vi "Test Run Asynchronous.vi"(11 "CO2 Settings":T3={"Run C1"={"A-1,  1"=inf, "A-3,  2"=inf, "A-4, 3"=9600.0, "A-5, 4"=8800.0, "ABCD-7, 5"=9800.0, "A-8, 6"=9800.0, "B-1,  7"=3400.0, "B-3, 8"=3400.0, "B-4,  9"=9600.0, "B-5, 10"=8800.0, "B-8, 11"=9800.0, "C-1, 12"=1800.0, "C-3, 13"=1800.0, "C-4, 14"=9600.0, "C-5,  15"=8800.0, "C-8, 16"=9800.0, "D-1, 17"=inf, "D-3, 18"=3400.0, "D-4,  19"=1800.0, "D-5,  20"=9800.0, "D-8,  21"=9800.0}, "Run C2"={"A-1,  1"=inf, "A-3,  2"=inf, "A-4, 3"=9500.0, "A-5, 4"=8600.0, "ABCD-7, 5"=9700.0, "A-8, 6"=9700.0, "B-1,  7"=3000.0, "B-3, 8"=3000.0, "B-4,  9"=9500.0, "B-5, 10"=8600.0, "B-8, 11"=9700.0, "C-1, 12"=1400.0, "C-3, 13"=1400.0, "C-4, 14"=9500.0, "C-5,  15"=8600.0, "C-8, 16"=9700.0, "D-1, 17"=inf, "D-3, 18"=3000.0, "D-4,  19"=1400.0, "D-5,  20"=9700.0, "D-8,  21"=9700.0}, "Hold C3"={"A-1,  1"=1800.0, "A-3,  2"=1800.0, "A-4, 3"=9000.0, "A-5, 4"=8800.0, "ABCD-7, 5"=9800.0, "A-8, 6"=9800.0, "B-1,  7"=3400.0, "B-3, 8"=3400.0, "B-4,  9"=9000.0, "B-5, 10"=8800.0, "B-8, 11"=9800.0, "C-1, 12"=1800.0, "C-3, 13"=1800.0, "C-4, 14"=9000.0, "C-5,  15"=8800.0, "C-8, 16"=9800.0, "D-1, 17"=1800.0, "D-3, 18"=3400.0, "D-4,  19"=1800.0, "D-5,  20"=9800.0, "D-8,  21"=9800.0}, "Hold C4"={"A-1,  1"=1400.0, "A-3,  2"=1400.0, "A-4, 3"=8800.0, "A-5, 4"=8600.0, "ABCD-7, 5"=9700.0, "A-8, 6"=9700.0, "B-1,  7"=3000.0, "B-3, 8"=3000.0, "B-4,  9"=8800.0, "B-5, 10"=8600.0, "B-8, 11"=9700.0, "C-1, 12"=1400.0, "C-3, 13"=1400.0, "C-4, 14"=8800.0, "C-5,  15"=8600.0, "C-8, 16"=9700.0, "D-1, 17"=1400.0, "D-3, 18"=3000.0, "D-4,  19"=1400.0, "D-5,  20"=9700.0, "D-8,  21"=9700.0}, "High CO2 Forces"={"A-1, 1"=TRUE, "A-3, 2"=TRUE, "A-4, 3"=FALSE, "A-5, 4"=TRUE, "ABCD-7, 5"=FALSE, "A-8, 6"=TRUE, "B-1,  7"=TRUE, "B-3, 8"=TRUE, "B-4, 9"=FALSE, "B-5, 10"=TRUE, "B-8,  11"=TRUE, "C-1, 12"=TRUE, "C-3, 13"=TRUE, "C-4,  14"=FALSE, "C-5,  15"=TRUE, "C-8, 16"=TRUE, "D-1, 17"=TRUE, "D-3, 18"=TRUE, "D-4, 19"=TRUE, "D-5,  20"=TRUE, "D-8,  21"=TRUE}}) -> ()   [LabVIEW 2012]
uses:
  Type Defs/AD Settings.ctl
  Type Defs/Output Values.ctl
  Type Defs/Output Switches.ctl
  Type Defs/CO2 Settings.ctl
  Type Defs/Final Output for Dispaly 2.ctl
panel:
  in  "Main Tabs":T1(tab)=enum."CO2 Settings"
  in  "Other Outputs":cluster{"Alarm":bool, "Heater":bool}
  out "CO2 ppm":u32(slide)=493 scale=0.0..10000.0
  out "Alt Dif":dbl(slide)=1604.2180978990014 scale=-1000.0..1000.0 scale format="%.1f"
  out "Final Output":T2
  in  "AD Settings":T6={"Set Point Force"={"A-1,  1"=inf, "A-3,  2"=inf, "A-4, 3"=inf, "A-5, 4"=5790.0, "ABCD-7, 5"=inf, "A-8, 6"=inf, "B-1,  7"=5790.0, "B-3, 8"=5790.0, "B-4,  9"=inf, "B-5, 10"=5790.0, "B-8, 11"=inf, "C-1, 12"=inf, "C-3, 13"=inf, "C-4, 14"=inf, "C-5,  15"=5790.0, "C-8, 16"=inf, "D-1, 17"=inf, "D-3, 18"=inf, "D-4,  19"=inf, "D-5,  20"=inf, "D-8,  21"=inf}, "Run A1"={"A-1,  1"=inf, "A-3,  2"=inf, "A-4, 3"=3.0, "A-5, 4"=inf, "ABCD-7, 5"=67.0, "A-8, 6"=630.0, "B-1,  7"=-30.0, "B-3, 8"=-30.0, "B-4,  9"=3.0, "B-5, 10"=inf, "B-8, 11"=630.0, "C-1, 12"=-60.0, "C-3, 13"=-60.0, "C-4, 14"=3.0, "C-5,  15"=inf, "C-8, 16"=630.0, "D-1, 17"=inf, "D-3, 18"=-30.0, "D-4,  19"=-60.0, "D-5,  20"=630.0, "D-8,  21"=930.0}, "Run A2"={"A-1,  1"=inf, "A-3,  2"=inf, "A-4, 3"=-3.0, "A-5, 4"=inf, "ABCD-7, 5"=60.0, "A-8, 6"=610.0, "B-1,  7"=-100.0, "B-3, 8"=-100.0, "B-4,  9"=-3.0, "B-5, 10"=inf, "B-8, 11"=610.0, "C-1, 12"=-120.0, "C-3, 13"=-120.0, "C-4, 14"=-3.0, "C-5,  15"=inf, "C-8, 16"=610.0, "D-1, 17"=inf, "D-3, 18"=-100.0, "D-4,  19"=-120.0, "D-5,  20"=610.0, "D-8,  21"=910.0}, "Hold A3"={"A-1,  1"=0.0, "A-3,  2"=0.0, "A-4, 3"=3.0, "A-5, 4"=inf, "ABCD-7, 5"=67.0, "A-8, 6"=630.0, "B-1,  7"=-150.0, "B-3, 8"=-150.0, "B-4,  9"=3.0, "B-5, 10"=inf, "B-8, 11"=630.0, "C-1, 12"=-300.0, "C-3, 13"=-300.0, "C-4, 14"=3.0, "C-5,  15"=inf, "C-8, 16"=630.0, "D-1, 17"=0.0, "D-3, 18"=-150.0, "D-4,  19"=-300.0, "D-5,  20"=630.0, "D-8,  21"=930.0}, "Hold A4"={"A-1,  1"=-150.0, "A-3,  2"=-150.0, "A-4, 3"=-3.0, "A-5, 4"=inf, "ABCD-7, 5"=60.0, "A-8, 6"=610.0, "B-1,  7"=-250.0, "B-3, 8"=-250.0, "B-4,  9"=-3.0, "B-5, 10"=inf, "B-8, 11"=610.0, "C-1, 12"=-500.0, "C-3, 13"=-500.0, "C-4, 14"=-3.0, "C-5,  15"=inf, "C-8, 16"=610.0, "D-1, 17"=-150.0, "D-3, 18"=-250.0, "D-4,  19"=-500.0, "D-5,  20"=610.0, "D-8,  21"=910.0}, "High AD Diff "={"A-1, 1"=FALSE, "A-3, 2"=FALSE, "A-4, 3"=FALSE, "A-5, 4"=TRUE, "ABCD-7, 5"=FALSE, "A-8, 6"=TRUE, "B-1,  7"=FALSE, "B-3, 8"=FALSE, "B-4, 9"=FALSE, "B-5, 10"=TRUE, "B-8,  11"=TRUE, "C-1, 12"=FALSE, "C-3, 13"=FALSE, "C-4,  14"=FALSE, "C-5,  15"=TRUE, "C-8, 16"=TRUE, "D-1, 17"=FALSE, "D-3, 18"=FALSE, "D-4, 19"=FALSE, "D-5,  20"=TRUE, "D-8,  21"=TRUE}, "Delay S"={"A-1,  1"=30.0, "A-3,  2"=30.0, "A-4, 3"=1.0, "A-5, 4"=1.0, "ABCD-7, 5"=1.0, "A-8, 6"=1.0, "B-1,  7"=30.0, "B-3, 8"=30.0, "B-4,  9"=1.0, "B-5, 10"=1.0, "B-8, 11"=1.0, "C-1, 12"=30.0, "C-3, 13"=30.0, "C-4, 14"=1.0, "C-5,  15"=1.0, "C-8, 16"=1.0, "D-1, 17"=30.0, "D-3, 18"=30.0, "D-4,  19"=30.0, "D-5,  20"=1.0, "D-8,  21"=1.0}}
  # "Channel A"
  # "Channel B"
  # "Channel C"
  # "Channel D"
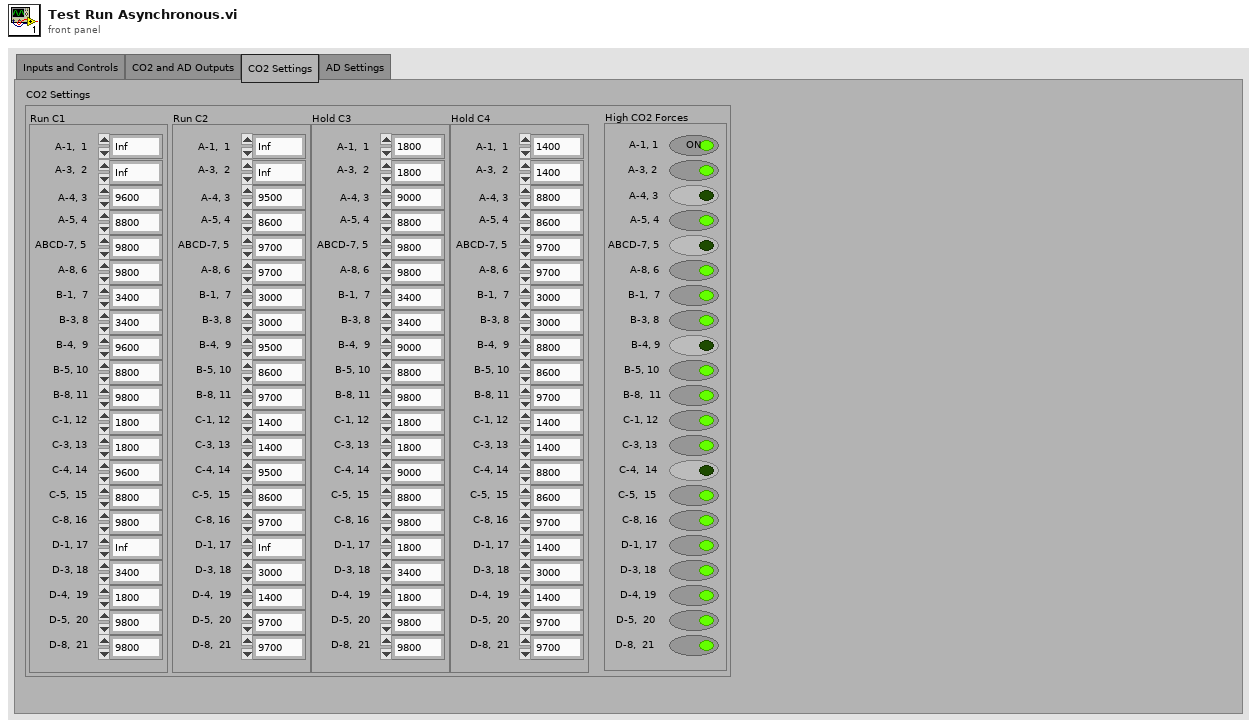
[diagram p1: front panel]
types:
  T1 = enum32{"Inputs and Controls", "CO2 and AD Outputs", "CO2 Settings", "AD Settings"}
  T2 = typedef "Final Output for Dispaly 2.ctl" = cluster{"A-1,  1":bool, "A-3,  2":bool, "A-4, 3":bool, "A-5, 4":bool, "ABCD-7, 5":bool, "A-8, 6":bool, "B-1,  7":bool, "B-3, 8":bool, "B-4,  9":bool, "B-5, 10":bool, "B-8, 11":bool, "C-1, 12":bool, "C-3, 13":bool, "C-4, 14":bool, "C-5,  15":bool, "C-8, 16":bool, "D-1, 17":bool, "D-3, 18":bool, "D-4,  19":bool, "D-5,  20":bool, "D-8,  21":bool}
  T3 = typedef "CO2 Settings.ctl" = cluster{"Run C1":T4, "Run C2":T4, "Hold C3":T4, "Hold C4":T4, "High CO2 Forces":T5}
  T4 = typedef "Output Values.ctl" = cluster{"A-1,  1":dbl, "A-3,  2":dbl, "A-4, 3":dbl, "A-5, 4":dbl, "ABCD-7, 5":dbl, "A-8, 6":dbl, "B-1,  7":dbl, "B-3, 8":dbl, "B-4,  9":dbl, "B-5, 10":dbl, "B-8, 11":dbl, "C-1, 12":dbl, "C-3, 13":dbl, "C-4, 14":dbl, "C-5,  15":dbl, "C-8, 16":dbl, "D-1, 17":dbl, "D-3, 18":dbl, "D-4,  19":dbl, "D-5,  20":dbl, "D-8,  21":dbl}
  T5 = typedef "Output Switches.ctl" = cluster{"A-1, 1":bool, "A-3, 2":bool, "A-4, 3":bool, "A-5, 4":bool, "ABCD-7, 5":bool, "A-8, 6":bool, "B-1,  7":bool, "B-3, 8":bool, "B-4, 9":bool, "B-5, 10":bool, "B-8,  11":bool, "C-1, 12":bool, "C-3, 13":bool, "C-4,  14":bool, "C-5,  15":bool, "C-8, 16":bool, "D-1, 17":bool, "D-3, 18":bool, "D-4, 19":bool, "D-5,  20":bool, "D-8,  21":bool}
  T6 = typedef "AD Settings.ctl" = cluster{"Set Point Force":T4, "Run A1":T4, "Run A2":T4, "Hold A3":T4, "Hold A4":T4, "High AD Diff ":T5, "Delay S":T4}
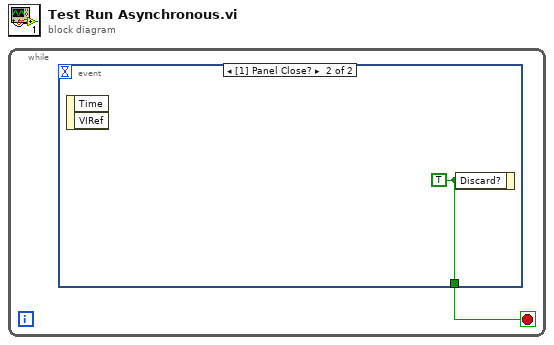
[diagram p0: block diagram]
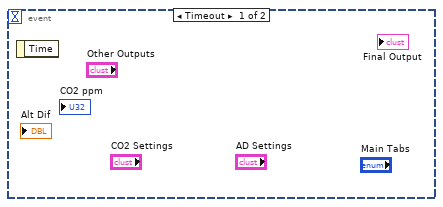
[diagram p2: hidden frame]
diagram:
  n1 = while {
    stop <- w1 stop-if-true
    n2 = event shown="[1] Panel Close?" {
      selector: _ -> [_ _]
      dyn-events: _ -> [_ _]
      timeout: _ -> [_ _]
      tunnel: [_ w2] -> w1
      event Timeout {
        n3 = event-data() -> ()  [unwired: 1 in, 1 out]
      }
      event Panel Close? {
        w2 = TRUE ("Discard?")
        n4 = event-data() -> ()  [unwired: 1 in, 2 out]
        n5 = event-data("Discard?"=w2) -> ()  [unwired: 1 in, 1 out]
      }
    }
  }
